vi "telemetria2.vi"(11 "Output Array":string[][](array[string])) -> (0 "ŚREDNIE NAPEDY":T3, 2 "output 1000 Lewy":cluster{"ERROR":dbl, i16}, 3 "out 100 prawy":cluster{"ERROR2":dbl, u16}, 7 "MANIPULATOR wy":T1, 8 "RAW NAPEDY":T2)   [LabVIEW 2015]
uses:
  <vilib>/ptbypt/NI_PtbyPt.lvlib
panel:
  out "Prad Prawy":cluster{u16}(graph)
  out "Prad Lewy":cluster{i16}(graph)
  out "ERROR Prawy":u16(graph)
  out "PIOUT Prawy":cluster{u16}(graph)
  out "match + rest of string":string
  out "substring before match":string
  out "concatenated string":string
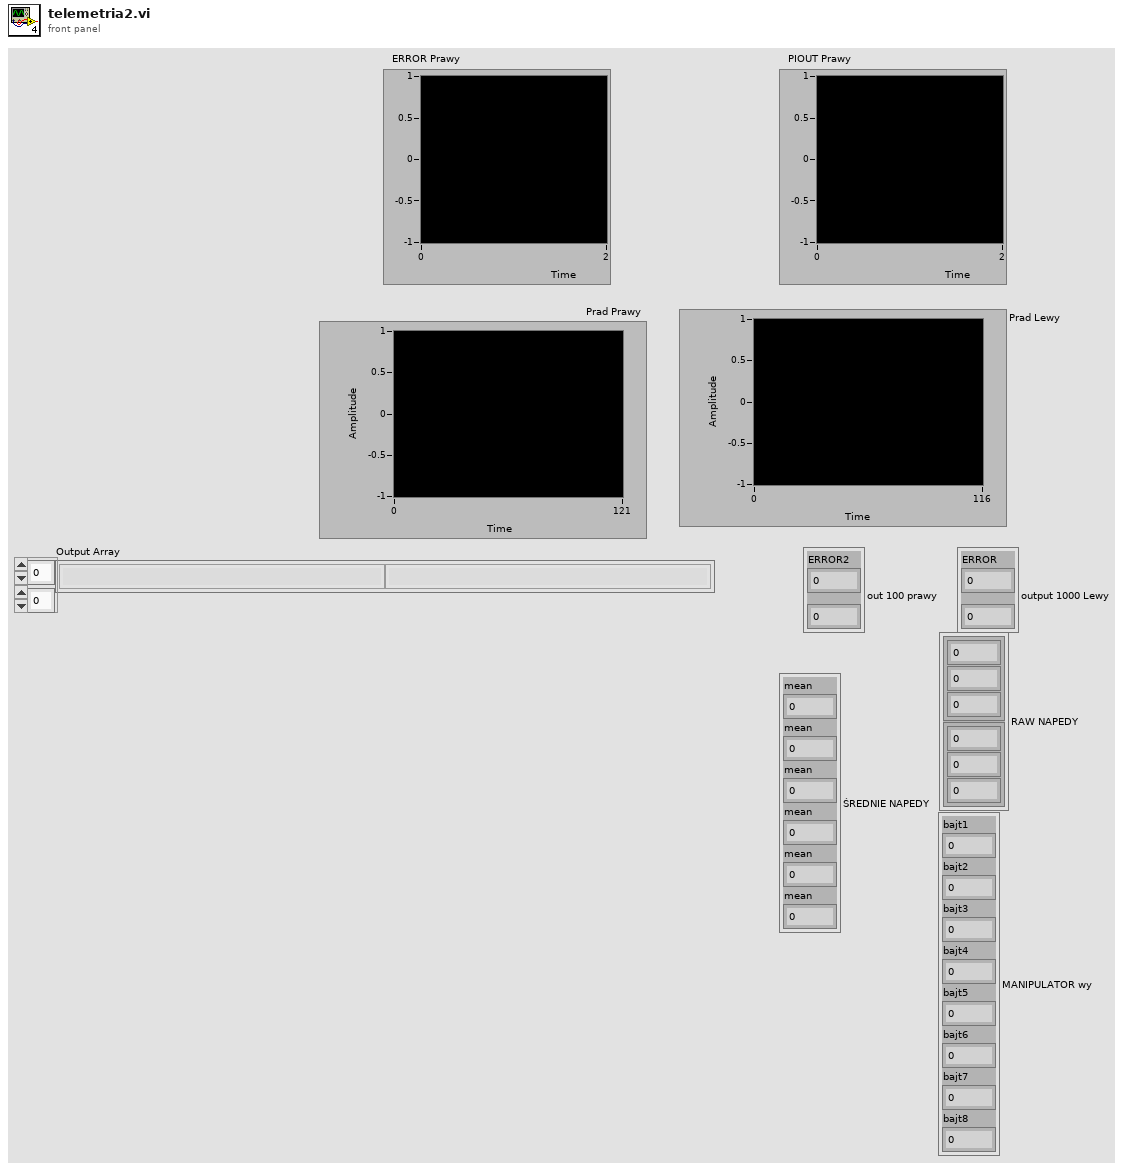
[diagram p1: front panel]
types:
  T1 = cluster{"bajt1":u8, "bajt2":u8, "bajt3":u8, "bajt4":u8, "bajt5":u8, "bajt6":u8, "bajt7":u8, "bajt8":u8}
  T2 = cluster{cluster{i16, i16, i16}, cluster{i16, i16, i16}}
  T3 = cluster{"mean":dbl, "mean":dbl, "mean":dbl, "mean":dbl, "mean":dbl, "mean":dbl}
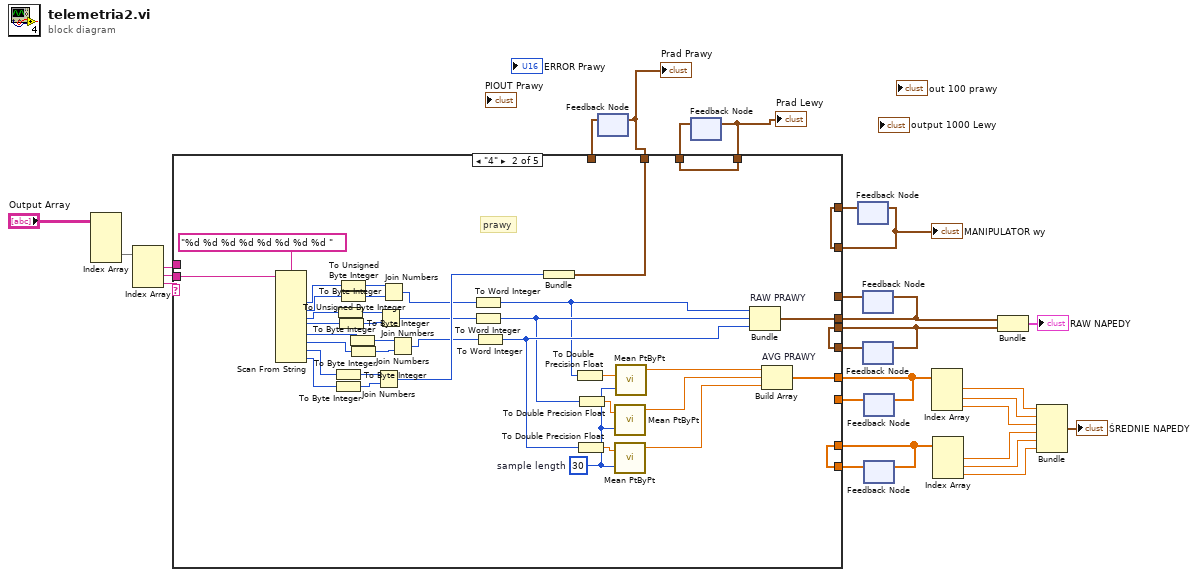
[diagram p0: block diagram]
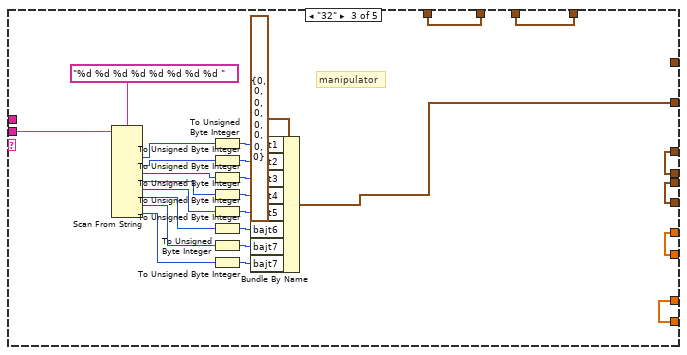
[diagram p3: hidden frame]
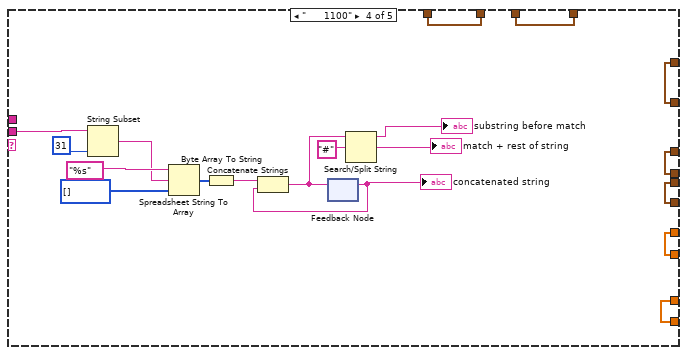
[diagram p4: hidden frame]
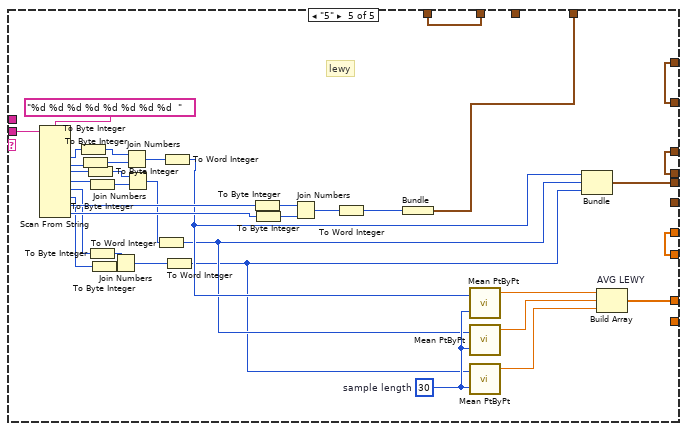
[diagram p5: hidden frame]
diagram:
  n1 = Index Array(array="Output Array") -> (element #2=w26:string[])  [unwired: 4 in, 1 out]
  n2 = Index Array(array=w26) -> (element #1=w22:string, element #2=w25:string, element #3=w24:string)  [unwired: 3 in]
  n3 = feedback #1() -> (w4:cluster{u16})  [unwired: 1 in]
  n4 = feedback #2() -> (w3:cluster{i16})  [unwired: 1 in]
  n5 = feedback #3() -> (w5:T1)  [unwired: 1 in]
  n6 = feedback #4() -> (w16:cluster{i16, i16, i16})  [unwired: 1 in]
  n7 = feedback #5() -> (w18:cluster{i16, i16, i16})  [unwired: 1 in]
  n8 = feedback #6() -> (w23:dbl[])  [unwired: 1 in]
  n9 = feedback #7() -> (w21:dbl[])  [unwired: 1 in]
  n10 = case shown="\"4\"" w24 {
    tunnel: w25 -> [_ w72 w98 w115 w154]
    tunnel: w23 -> [w31 _ w94 w104 w147]
    tunnel: w22 -> [_ _ _ _ _]
    tunnel: [w34 w71 w97 w118 w143] -> w11
    tunnel: w21 -> [w34 w71 w97 w118 _]
    tunnel: [w28 w35 w74 w100 w142] -> w2
    tunnel: [w29 w70 w75 w101 w119] -> w1
    tunnel: [w32 w62 w95 w105 w148] -> w17
    tunnel: [w33 w61 w96 w106 w149] -> w19
    tunnel: w18 -> [w33 w61 w96 w106 _]
    tunnel: w16 -> [w32 _ w95 w105 w148]
    tunnel: [w31 w57 w94 w104 w147] -> w12
    tunnel: [w30 w36 w76 w102 w120] -> w6
    tunnel: w5 -> [w30 w36 _ w102 w120]
    tunnel: w4 -> [w29 _ w75 w101 w119]
    tunnel: w3 -> [w28 w35 w74 w100 _]
    frame "False", Default {
    }
    frame "4" {
      w44 = 30  # sample length
      # "prawy"
      n11 = Scan From String(format string="%d %d %d %d %d %d %d %d ", input string=w72) -> (output 1=w47:i32, output 2=w48:i32, output 3=w49:i32, output 4=w50:i32, output 5=w51:i32, output 6=w52:i32, output 7=w69:i32, output 8=w68:i32)  [unwired: 10 in, 3 out]
      n12 = To Byte Integer(number=w69) -> (8bit integer=w67:i8)
      n13 = To Byte Integer(number=w68) -> (8bit integer=w66:i8)
      n14 = To Byte Integer(number=w49) -> (8bit integer=w55:i8)
      n15 = To Byte Integer(number=w50) -> (8bit integer=w56:i8)
      n16 = To Unsigned Byte Integer(number=w47) -> (unsigned 8bit integer=w64:u8)
      n17 = To Unsigned Byte Integer(number=w48) -> (unsigned 8bit integer=w63:u8)
      n18 = To Byte Integer(number=w51) -> (8bit integer=w54:i8)
      n19 = To Byte Integer(number=w52) -> (8bit integer=w53:i8)
      n20 = Join Numbers(hi=w67, lo=w66) -> ((hi.lo)=w65:u16)
      n21 = Join Numbers(hi=w55, lo=w56) -> ((hi.lo)=w45:u16)
      n22 = Join Numbers(hi=w64, lo=w63) -> ((hi.lo)=w46:u16)
      n23 = Join Numbers(hi=w54, lo=w53) -> ((hi.lo)=w40:u16)
      n24 = To Word Integer(number=w46) -> (16bit integer=w37:i16)
      n25 = To Word Integer(number=w45) -> (16bit integer=w38:i16)
      n26 = To Word Integer(number=w40) -> (16bit integer=w39:i16)
      n27 = Bundle(w65) -> (w70:cluster{u16})  [unwired: 1 in]
      n28 = To Double Precision Float(number=w37) -> (double precision float=w43:dbl)
      n29 = To Double Precision Float(number=w39) -> (double precision float=w41:dbl)
      n30 = To Double Precision Float(number=w38) -> (double precision float=w42:dbl)
      n31 = call <vilib>:"Mean PtByPt.vi"("x"=w42, "sample length"=w44) -> ("mean"=w59:dbl)  [unwired: 2 in, 1 out]
      n32 = call <vilib>:"Mean PtByPt.vi"("x"=w41, "sample length"=w44) -> ("mean"=w58:dbl)  [unwired: 2 in, 1 out]
      n33 = call <vilib>:"Mean PtByPt.vi"("x"=w43, "sample length"=w44) -> ("mean"=w60:dbl)  [unwired: 2 in, 1 out]
      n34 = Bundle "RAW PRAWY"(w37, w38, w39) -> (w62:cluster{i16, i16, i16})  [unwired: 1 in]
      n35 = Build Array "AVG PRAWY"(w60, w59, w58) -> (w57:dbl[])
    }
    frame "32" {
      # "manipulator"
      n36 = Scan From String(format string="%d %d %d %d %d %d %d %d ", input string=w98) -> (output 1=w93:i32, output 2=w92:i32, output 3=w91:i32, output 4=w90:i32, output 5=w89:i32, output 6=w88:i32, output 7=w87:i32, output 8=w86:i32)  [unwired: 10 in, 3 out]
      n37 = To Unsigned Byte Integer(number=w93) -> (unsigned 8bit integer=w84:u8)
      n38 = To Unsigned Byte Integer(number=w92) -> (unsigned 8bit integer=w83:u8)
      n39 = To Unsigned Byte Integer(number=w91) -> (unsigned 8bit integer=w82:u8)
      n40 = To Unsigned Byte Integer(number=w90) -> (unsigned 8bit integer=w81:u8)
      n41 = To Unsigned Byte Integer(number=w89) -> (unsigned 8bit integer=w80:u8)
      n42 = To Unsigned Byte Integer(number=w88) -> (unsigned 8bit integer=w79:u8)
      n43 = To Unsigned Byte Integer(number=w87) -> (unsigned 8bit integer=w78:u8)
      n44 = To Unsigned Byte Integer(number=w86) -> (unsigned 8bit integer=w77:u8)
      n45 = Bundle By Name(cluster=T1 {"bajt1"=0, "bajt2"=0, "bajt3"=0, "bajt4"=0, "bajt5"=0, "bajt6"=0, "bajt7"=0, "bajt8"=0} ("MANIPULATOR can"), "bajt1"=w84, "bajt2"=w83, "bajt3"=w82, "bajt4"=w81, "bajt5"=w80, "bajt6"=w79, "bajt7"=w78, "bajt7"=w77) -> (w76:T1)
    }
    frame "      1100" {
      n46 = String Subset(string=w115, length (rest)=31 ("length (rest)")) -> (substring=w113:string)  [unwired: 1 in]
      n47 = Spreadsheet String To Array(format string="%s", spreadsheet string=w113, array type (2D Dbl)=u8[] [] ("unsigned byte array")) -> (array=w112:u8[])  [unwired: 1 in]
      n48 = Byte Array To String(unsigned byte array=w112) -> (string=w107:string)
      n49 = feedback #8() -> (w111:string)  [unwired: 1 in]
      "concatenated string" <- w111
      n50 = Concatenate Strings(w107, w111) -> (w110:string)
      n51 = feedback-in #8(w110) -> ()
      n52 = Search/Split String(string=w110, search string/char (-)="#") -> (substring before match=→"substring before match":string, match + rest of string=→"match + rest of string":string)  [unwired: 1 in, 1 out]
    }
    frame "5" {
      w123 = 30  # sample length
      # "lewy"
      n53 = Scan From String(format string="%d %d %d %d %d %d %d %d  ", input string=w154) -> (output 1=w138:i32, output 2=w137:i32, output 3=w132:i32, output 4=w134:i32, output 5=w131:i32, output 6=w130:i32, output 7=w152:i32, output 8=w150:i32)  [unwired: 10 in, 3 out]
      n54 = To Byte Integer(number=w138) -> (8bit integer=w133:i8)
      n55 = To Byte Integer(number=w137) -> (8bit integer=w139:i8)
      n56 = To Byte Integer(number=w132) -> (8bit integer=w136:i8)
      n57 = To Byte Integer(number=w134) -> (8bit integer=w135:i8)
      n58 = To Byte Integer(number=w131) -> (8bit integer=w129:i8)
      n59 = To Byte Integer(number=w130) -> (8bit integer=w128:i8)
      n60 = Join Numbers(hi=w129, lo=w128) -> ((hi.lo)=w125:u16)
      n61 = Join Numbers(hi=w133, lo=w139) -> ((hi.lo)=w127:u16)
      n62 = Join Numbers(hi=w136, lo=w135) -> ((hi.lo)=w124:u16)
      n63 = To Word Integer(number=w124) -> (16bit integer=w122:i16)
      n64 = To Word Integer(number=w127) -> (16bit integer=w126:i16)
      n65 = To Word Integer(number=w125) -> (16bit integer=w121:i16)
      n66 = To Byte Integer(number=w152) -> (8bit integer=w153:i8)
      n67 = To Byte Integer(number=w150) -> (8bit integer=w151:i8)
      n68 = Join Numbers(hi=w153, lo=w151) -> ((hi.lo)=w140:u16)
      n69 = To Word Integer(number=w140) -> (16bit integer=w141:i16)
      n70 = Bundle(w141) -> (w142:cluster{i16})  [unwired: 1 in]
      n71 = call <vilib>:"Mean PtByPt.vi"("x"=w126, "sample length"=w123) -> ("mean"=w146:dbl)  [unwired: 2 in, 1 out]
      n72 = call <vilib>:"Mean PtByPt.vi"("x"=w122, "sample length"=w123) -> ("mean"=w145:dbl)  [unwired: 2 in, 1 out]
      n73 = call <vilib>:"Mean PtByPt.vi"("x"=w121, "sample length"=w123) -> ("mean"=w144:dbl)  [unwired: 2 in, 1 out]
      n74 = Bundle ("RAW LEWY")(w126, w122, w121) -> (w149:cluster{i16, i16, i16})  [unwired: 1 in]
      n75 = Build Array "AVG LEWY"(w146, w145, w144) -> (w143:dbl[])
    }
  }
  "Prad Lewy" <- w2
  "Prad Prawy" <- w1
  "MANIPULATOR wy" <- w6
  n76 = feedback-in #1(w1) -> ()
  n77 = feedback-in #2(w2) -> ()
  n78 = feedback-in #3(w6) -> ()
  n79 = feedback-in #4(w17) -> ()
  n80 = feedback-in #5(w19) -> ()
  n81 = feedback-in #6(w12) -> ()
  n82 = feedback-in #7(w11) -> ()
  n83 = Index Array(array=w12) -> (element #1=w15:dbl, element #2=w14:dbl, element #3=w13:dbl)  [unwired: 3 in]
  n84 = Index Array(array=w11) -> (element #1=w10:dbl, element #2=w9:dbl, element #3=w8:dbl)  [unwired: 3 in]
  n85 = Bundle ("RAW NAPEDY")(w17, w19) -> (→"RAW NAPEDY":T2)  [unwired: 1 in]
  n86 = Bundle("mean"=w15, "mean"=w14, "mean"=w13, "mean"=w10, "mean"=w9, "mean"=w8) -> (→"ŚREDNIE NAPEDY":T3)  [unwired: 1 in]
